vi "Button2Toggle.vi"(10 "Boolean":bool) -> (0 "changed?":bool, 2 "Latched Boolean":bool)   [LabVIEW 2011]
uses:
  <vilib>/ptbypt/NI_PtbyPt.lvlib
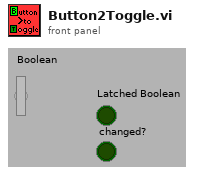
[diagram p1: front panel]
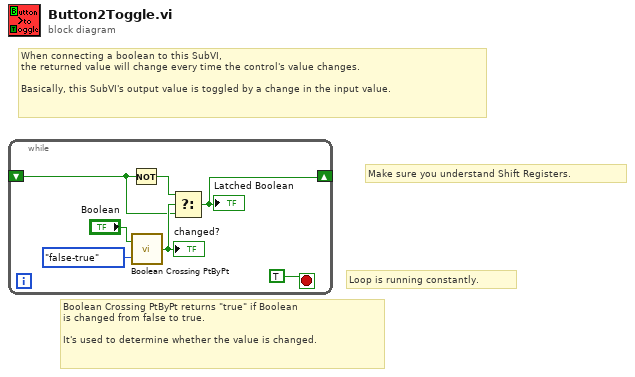
[diagram p0: block diagram]
diagram:
  # "Boolean Crossing PtByPt returns \"true\" if Boolean\nis changed from false to true.\n\nIt's used to determine whether the value is changed."
  # "Loop is running constantly."
  # "Make sure you understand Shift Registers."
  # "When connecting a boolean to this SubVI,\nthe returned value will change every time the control's value changes.\n\nBasically, this SubVI's output value is toggled by a change in the input value."
  n1 = while {
    shift-right: [w3] -> _
    shift-left: _ -> [w2]
    stop <- TRUE stop-if-true
    n2 = Not(x=w2) -> (.not. x?=w4:bool)
    n3 = call <vilib>:"Boolean Crossing PtByPt.vi"("direction"=enum16{"either", "false-true", "true-false"}."false-true", "input"="Boolean") -> ("crossing"=w6:bool)  [unwired: 1 in]
    "changed?" <- w6
    n4 = Select(t=w4, s=w6, f=w2) -> (s? t:f=w3:bool)
    "Latched Boolean" <- w3
  }
